vi "TcA07-001_ObjectStatusInformation.vi"(1 "Input buffer":T3="1", 3 "Invocation info":T2, 5 "error in (no error)":errorcluster, 6 "Add log to result?":bool) -> (16 "Test Data":T1 {"Numeric Measurement" format="%.2f"}, 19 "error out":errorcluster)   [LabVIEW 2020]
doc: "Test case template."
uses:
  Shared/Support_InputBuffer.ctl
  Shared/Support_InvocationInfo.ctl
  Shared/Support_TestData.ctl
  TestClasses/G#SubClass1_class/G#SubClass1.lvclass
  <vilib>/addons/_AddQ/G#Object/G#Object.lvclass
panel:
  in  "Test name":string="TcA07-001 Object status information"
  out "Test result":bool
  out "Result":string
  # "Verify that the object status information method returns the\ncorrect information about the object."
  # "Sub test case"
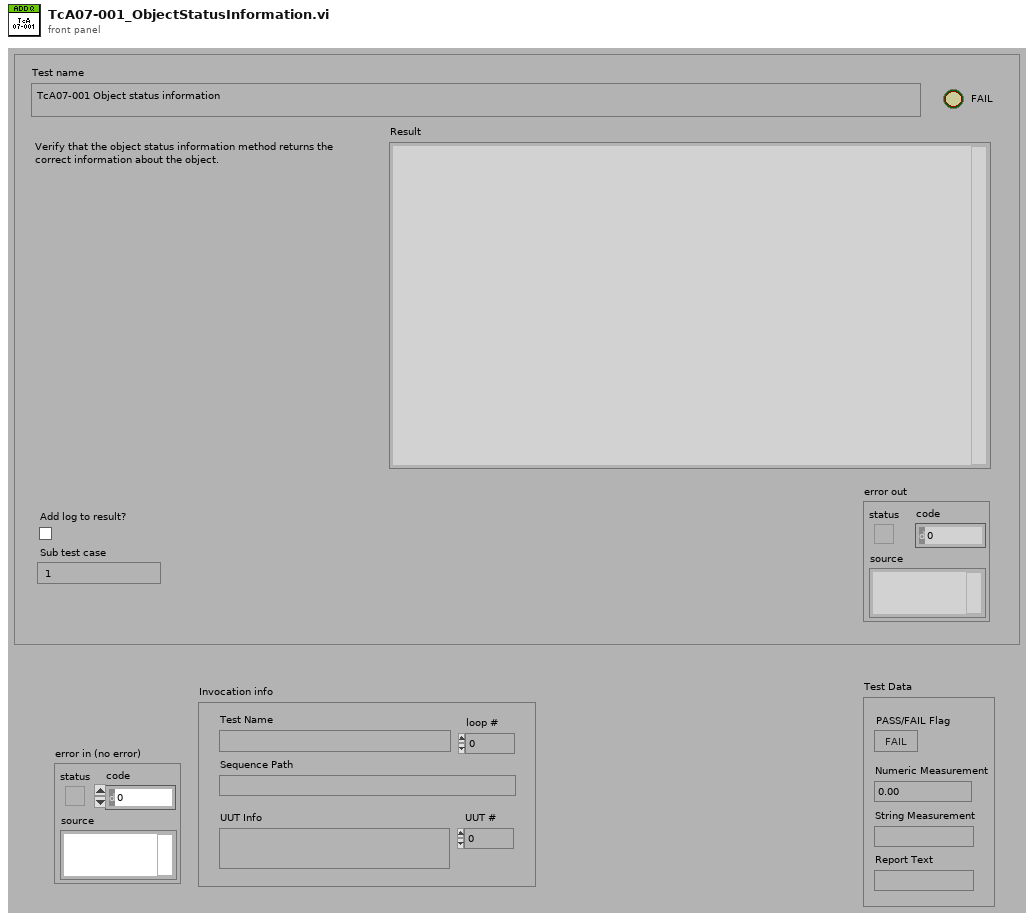
[diagram p1: front panel]
types:
  T1 = typedef "Support_TestData.ctl" = cluster{"PASS/FAIL Flag":bool, "Numeric Measurement":dbl, "String Measurement":string, "Report Text":string}
  T2 = typedef "Support_InvocationInfo.ctl" = cluster{"UUT #":i32, "loop #":i32, "UUT Info":string, "Test Name":string, "Sequence Path":path}
  T3 = typedef "Support_InputBuffer.ctl" = string
  T4 = typedef "Support_ResultType.ctl" = cluster{"Pass":bool, "Comment":string, "MeasurementValue":dbl}
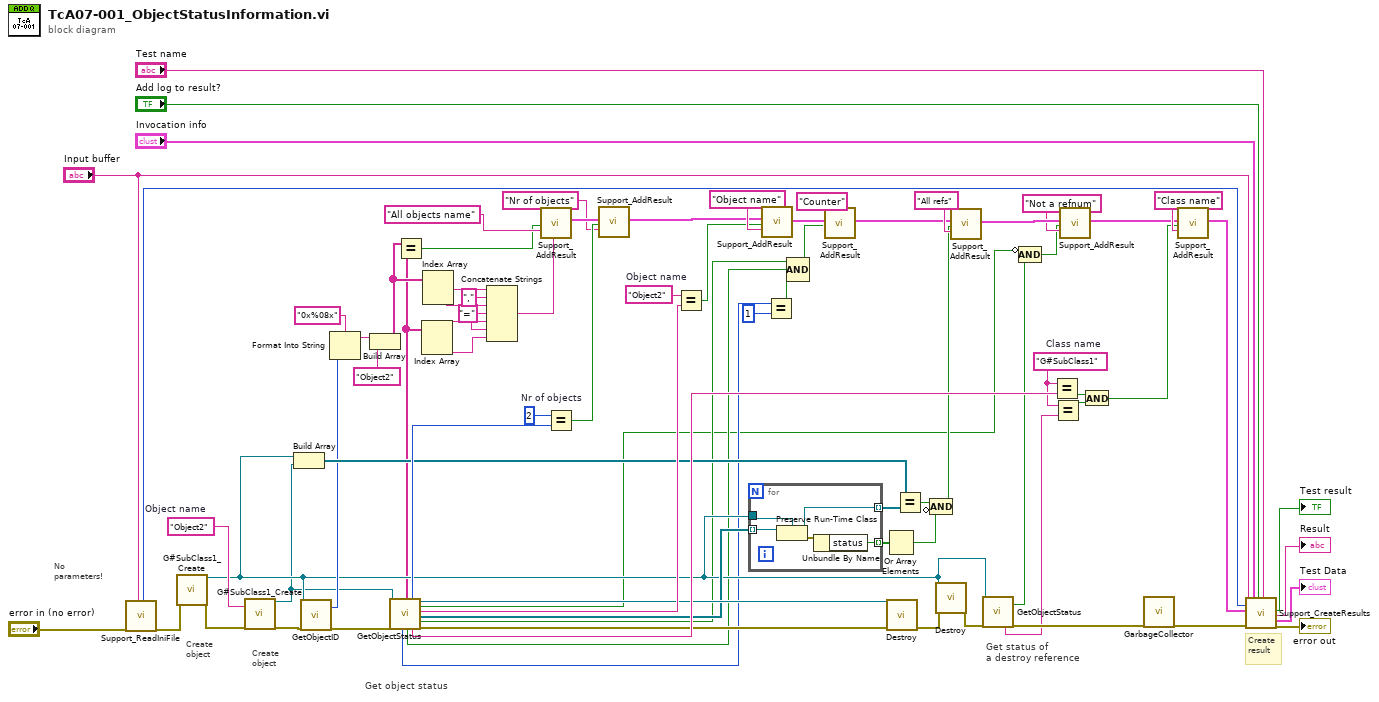
[diagram p0: block diagram]
diagram:
  w13 = "," ("string")
  w63 = 2  # Nr of objects
  w64 = "Object2"  # Object name
  w4 = "G#SubClass1"  # Class name
  w65 = "Object2"  # Object name
  # "Create\nobject"
  # "Create\nobject"
  # "Get status of\na destroy reference"
  # "Get object status"
  # "No\nparameters!"
  # "Create\nresult"
  n1 = call "Support_ReadIniFile.vi"("error in (no error)"="error in (no error)", "Sub test case"="Input buffer") -> ("Timer start"=w70:u32, "error out"=w47:errorcluster)  [unwired: 10 in, 6 out]
  n2 = call "G#SubClass1_Create.vi"("error in (no error)"=w47) -> ("reference out"=w50:refnum<class "G#SubClass1.lvclass">, "error out"=w69:errorcluster)  [unwired: 16 in, 1 out]
  n3 = call "G#SubClass1_Create.vi"("object name"=w65, "error in (no error)"=w69) -> ("reference out"=w49:refnum<class "G#SubClass1.lvclass">, "error out"=w10:errorcluster)  [unwired: 15 in, 1 out]
  n4 = Build Array(w50, w49) -> (w55:refnum<class "G#SubClass1.lvclass">[])
  n5 = call-dynamic "GetObjectID.vi"("reference in"=w50, "error in (no error)"=w10) -> ("object ID"=w53:u32, "error out"=w9:errorcluster)  [unwired: 15 in, 1 out]
  n6 = Format Into String(format string="0x%08x", w53) -> (resulting string=w52:string)  [unwired: 2 in, 1 out]
  n7 = Build Array(w52, "Object2") -> (w19:string[])
  n8 = call-dynamic "GetObjectStatus.vi"("reference in"=w49, "error in (no error)"=w9) -> ("# of users?"=w33:i32, "all object names"=w18:string[], "last user"=w36:bool, "# of objects"=w62:i32, "class name"=w60:string, "reference out"=w58:refnum<class "G#SubClass1.lvclass">, "not a refnum?"=w21:bool, "object name"=w61:string, "all refs out"=w57:refnum<class "G#Object.lvclass">[], "counter?"=w37:bool, "error out"=w59:errorcluster)  [unwired: 6 in, 1 out]
  n9 = Equal?(x=w19, y=w18) -> (x = y?=w45:bool)
  n10 = Index Array(array=w18) -> (element #1=w15:string, element #2=w14:string)  [unwired: 2 in]
  n11 = Index Array(array=w19) -> (element #1=w17:string, element #2=w16:string)  [unwired: 2 in]
  n12 = Concatenate Strings(w17, w13, w16, "=" ("string"), w15, w13, w14) -> (w11:string)
  n13 = call "Support_AddResult.vi"("Pass"=w45, "Comment"="All objects name", "Fail comment"=w11) -> ("Results out"=w44:T4[])  [unwired: 16 in]
  n14 = Equal?(x=w63, y=w62) -> (x = y?=w43:bool)
  n15 = call "Support_AddResult.vi"("Results in"=w44, "Pass"=w43, "Comment"="Nr of objects") -> ("Results out"=w20:T4[])  [unwired: 16 in]
  n16 = Equal?(x=w64, y=w61) -> (x = y?=w40:bool)
  n17 = for {
    tunnel: w57 -> [w84] mode=indexing
    tunnel: w50 -> [w83]
    tunnel: [w82] -> w56 mode=indexing
    tunnel: [w80] -> w31 mode=indexing
    n18 = Preserve Run-Time Class(object in=w84, 2:w83) -> (object out=w82:refnum<class "G#SubClass1.lvclass">, error out=w81:errorcluster)  [unwired: 1 in]
    n19 = Unbundle By Name(w81) -> ("status"=w80:bool)
  }
  n20 = call "Support_AddResult.vi"("Results in"=w20, "Pass"=w40, "Comment"="Object name") -> ("Results out"=w39:T4[])  [unwired: 16 in]
  n21 = Equal?(x=w33, y=1) -> (x = y?=w34:bool)
  n22 = Compound Arithmetic op=AND(w37, w36, w34) -> (w32:bool)
  n23 = call "Support_AddResult.vi"("Results in"=w39, "Pass"=w32, "Comment"="Counter") -> ("Results out"=w7:T4[])  [unwired: 16 in]
  n24 = Or Array Elements(Boolean array=w31) -> (logical OR=w29:bool)
  n25 = call-dynamic "Destroy.vi"("reference in"=w58, "error in (no error)"=w59) -> ("error out"=w68:errorcluster)  [unwired: 16 in, 1 out]
  n26 = Equal?(x=w55, y=w56) -> (x = y?=w30:bool)
  n27 = Compound Arithmetic op=AND(w30, invert w29) -> (w26:bool)
  n28 = call-dynamic "Destroy.vi"("reference in"=w50, "error in (no error)"=w68) -> ("error out"=w67:errorcluster)  [unwired: 16 in, 1 out]
  n29 = call "Support_AddResult.vi"("Results in"=w7, "Pass"=w26, "Comment"="All refs") -> ("Results out"=w25:T4[])  [unwired: 16 in]
  n30 = call-dynamic "GetObjectStatus.vi"("reference in"=w50, "error in (no error)"=w67) -> ("class name"=w8:string, "not a refnum?"=w23:bool, "error out"=w48:errorcluster)  [unwired: 6 in, 9 out]
  n31 = Compound Arithmetic op=AND(invert w21, w23) -> (w22:bool)
  n32 = Equal?(x=w4, y=w60) -> (x = y?=w3:bool)
  n33 = Equal?(x=w4, y=w8) -> (x = y?=w2:bool)
  n34 = call "Support_AddResult.vi"("Results in"=w25, "Pass"=w22, "Comment"="Not a refnum") -> ("Results out"=w6:T4[])  [unwired: 16 in]
  n35 = And(x=w3, y=w2) -> (x .and. y?=w1:bool)
  n36 = call <vilib>:"GarbageCollector.vi"("error in (no error)"=w48) -> ("error out"=w66:errorcluster)  [unwired: 16 in, 2 out]
  n37 = call "Support_AddResult.vi"("Results in"=w6, "Pass"=w1, "Comment"="Class name") -> ("Results out"=w5:T4[])  [unwired: 16 in]
  n38 = call "Support_CreateResults.vi"("Sub test case"="Input buffer", "Timer start"=w70, "Results"=w5, "error in (no error)"=w66, "Invocation info"="Invocation info", "Add log to result?"="Add log to result?", "Test name"="Test name") -> ("Pass/fail flag"=→"Test result":bool, "Result"=→"Result":string, "Test Data"=→"Test Data":T1, "error out"=→"error out":errorcluster)  [unwired: 9 in]
